vi "Camera_Snap_Jesse.vi"(8 "error in (no error)":errorcluster, 10 "Camera Session In":T1, 11 "Image In":T2) -> (0 "error out":errorcluster, 3 "New Image":T2)   [LabVIEW 2019]
uses:
  <vilib>/vision/Image Controls.llb/IMAQ Image.ctl
  <vilib>/userdefined/High Color/IMAQdx.ctl
  <vilib>/vision/driver/NI_Vision_Acquisition_Software.lvlib
panel:
  in  "CameraName":refnum<vi>
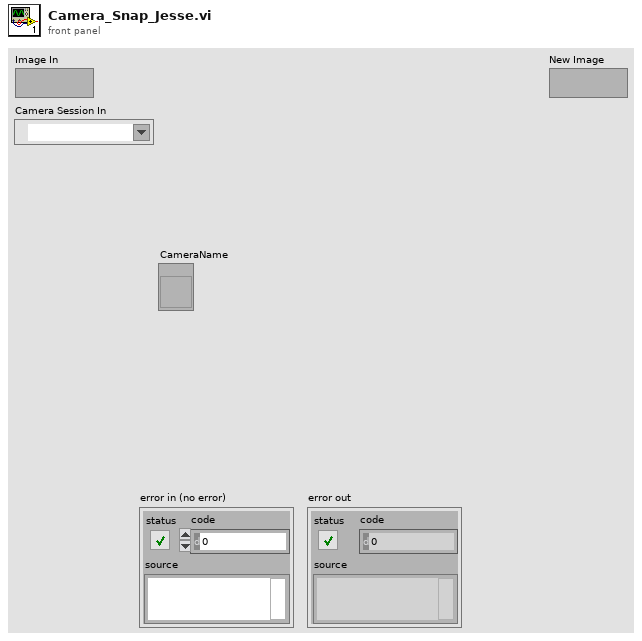
[diagram p1: front panel]
types:
  T1 = typedef "IMAQdx.ctl" = refnum<k21>
  T2 = typedef "IMAQ Image.ctl" = refnum<image>
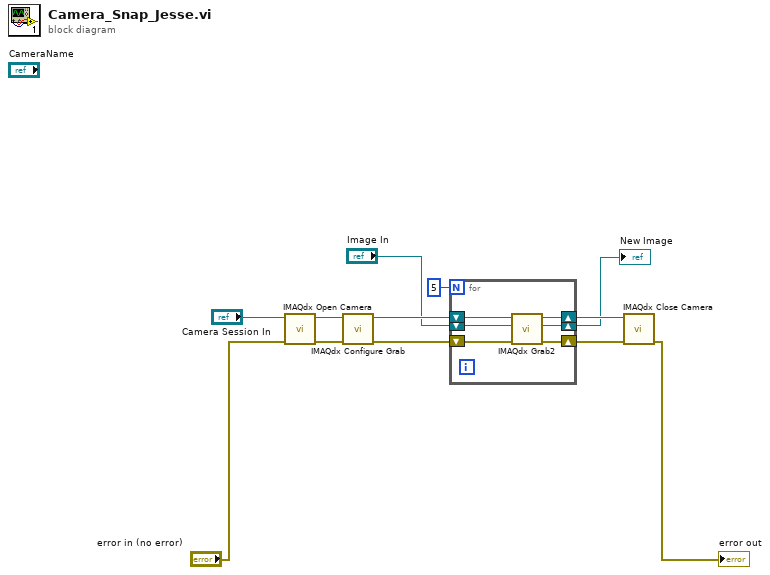
[diagram p0: block diagram]
diagram:
  n1 = call <vilib>:"IMAQdx Open Camera.vi"("error in"="error in (no error)", "Session In"="Camera Session In") -> ("error out"=w7:errorcluster, "Session Out"=w11:T1)  [unwired: 1 in, 7 out]
  n2 = call <vilib>:"IMAQdx Configure Grab.vi"("error in"=w7, "Session In"=w11) -> ("error out"=w6:errorcluster, "Session Out"=w8:T1)  [unwired: 8 in]
  n3 = for {
    N: 5 -> [_]
    shift-right: [w15] -> w9
    shift-left: "Image In" -> [w16]
    shift-right: [w18] -> w12
    shift-left: w8 -> [w14]
    shift-right: [w17] -> w10
    shift-left: w6 -> [w13]
    n4 = call <vilib>:"IMAQdx Grab2.vi"("error in"=w13, "Image In"=w16, "Session In"=w14) -> ("error out"=w17:errorcluster, "Image Out"=w15:T2, "Session Out"=w18:T1)  [unwired: 5 in, 1 out]
  }
  "New Image" <- w9
  n5 = call <vilib>:"IMAQdx Close Camera.vi"("error in"=w10, "Session In"=w12) -> ("error out"=→"error out":errorcluster)  [unwired: 9 out]
